vi "CmsInitializeQbus.vi"(8 "error in (no error)":errorcluster) -> (0 "error out":errorcluster, 3 "Qbus out":refnum<class "Qbus.lvclass">)   [LabVIEW 2017]
uses:
  <vilib>/addons/Qbus/Qbus.lvclass
  <vilib>/addons/BlinkProcess/BlinkProcess.lvlib
  <vilib>/addons/TimerProcess/TimerProcess.lvlib
  <vilib>/addons/InsightCM/Devices/Shared/Common/ServerComm/ServerComm.lvlib
  <vilib>/addons/InsightCM/Devices/Shared/Common/Trigger/Trigger.lvlib
  <vilib>/addons/InsightCM/Devices/Shared/Cms/CmsAnalysis/CmsAnalysis.lvlib
  <vilib>/addons/TraceLogger/TraceLogger.lvlib
  <vilib>/addons/InsightCM/Devices/Shared/Common/FileManager/FileManager.lvlib
  <vilib>/addons/InsightCM/Devices/Shared/Cms/CmsFpgaBitfileManager/CmsFpgaBitfileManager.lvlib
  <vilib>/addons/InsightCM/Devices/Shared/Common/Controller/Controller.lvlib
  <vilib>/addons/InsightCM/Devices/Shared/Common/DataAccumulator/DataAccumulator.lvlib
  <vilib>/addons/InsightCM/Devices/Shared/Common/DeviceHealth/DeviceHealth.lvlib
  <vilib>/addons/InsightCM/Devices/Shared/Common/SinglePointClock/SinglePointClock.lvlib
  <vilib>/addons/InsightCM/Devices/Shared/Cms/CmsVirtualChannel/CmsVirtualChannel.lvlib
  <vilib>/addons/InsightCM/Devices/Shared/Cms/CmsTestPanel/CmsTestPanel.lvlib
  <vilib>/addons/InsightCM/Devices/Shared/Common/ModbusMaster/ModbusMaster.lvlib
  <vilib>/addons/InsightCM/Devices/Shared/Cms/CmsDataEventCreator/CmsDataEventCreator.lvlib
  <vilib>/addons/InsightCM/Devices/Shared/Common/OpState/OpState.lvlib
  <vilib>/addons/InsightCM/Devices/Shared/Common/TrendAlarm/TrendAlarm.lvlib
  <vilib>/addons/InsightCM/Devices/Shared/Cms/CmsAnalysisHighRate/CmsAnalysisHighRate.lvlib
  <vilib>/addons/InsightCM/Devices/Shared/Cms/CmsAcquisition/CmsAcquisition.lvlib
  <vilib>/addons/InsightCM/Devices/Shared/Common/ScanEngine/ScanEngine.lvlib
  <vilib>/addons/InsightCM/Devices/Shared/Cms/CmsBurstMode/BurstMode.lvlib
  <vilib>/addons/InsightCM/Devices/Shared/Common/OPCUAClient/OPCUAClient.lvlib
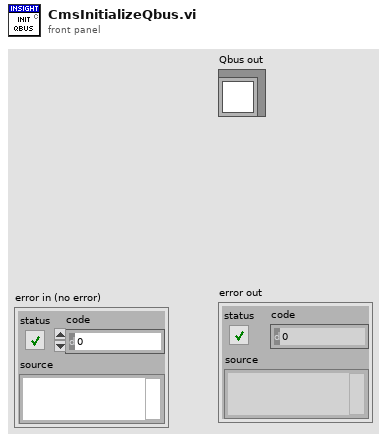
[diagram p1: front panel]
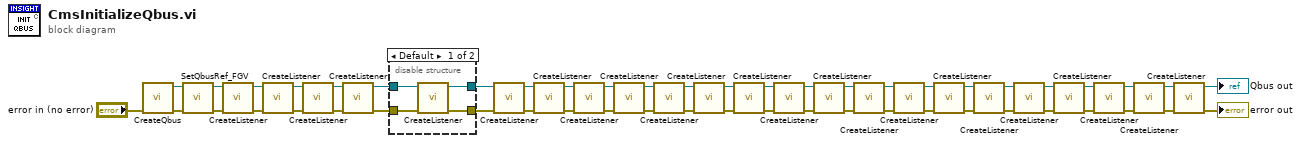
[diagram p0: block diagram]
diagram:
  n1 = call <vilib>:"CreateQbus.vi"("error in (no error)"="error in (no error)") -> ("error out"=w44:errorcluster, "Qbus"=w43:refnum<class "Qbus.lvclass">)  [unwired: 9 in]
  n2 = call <vilib>:"SetQbusRef_FGV.vi"("error in (no error)"=w44, "Qbus in"=w43) -> ("error out"=w42:errorcluster, "Qbus out"=w41:refnum<class "Qbus.lvclass">)  [unwired: 8 in]
  n3 = call <vilib>:"CreateListener.vi"("error in (no error)"=w42, "Qbus in"=w41) -> ("error out"=w46:errorcluster, "Qbus out"=w45:refnum<class "Qbus.lvclass">)  [unwired: 8 in]
  n4 = call <vilib>:"CreateListener.vi"("error in (no error)"=w46, "Qbus in"=w45) -> ("error out"=w33:errorcluster, "Qbus out"=w34:refnum<class "Qbus.lvclass">)  [unwired: 8 in]
  n5 = call <vilib>:"CreateListener.vi"("error in (no error)"=w33, "Qbus in"=w34) -> ("error out"=w32:errorcluster, "Qbus out"=w31:refnum<class "Qbus.lvclass">)  [unwired: 8 in]
  n6 = call <vilib>:"CreateListener.vi"("error in (no error)"=w32, "Qbus in"=w31) -> ("error out"=w2:errorcluster, "Qbus out"=w4:refnum<class "Qbus.lvclass">)  [unwired: 8 in]
  n7 = disable-structure shown="Default" {
    disable-tunnel: w4 -> [w55 w57]
    disable-tunnel: [w54 w57] -> w3
    disable-tunnel: w2 -> [w53 w56]
    disable-tunnel: [w52 w56] -> w1
    frame condition #0 (active) {
      n8 = call <vilib>:"CreateListener.vi"("error in (no error)"=w53, "Qbus in"=w55) -> ("error out"=w52:errorcluster, "Qbus out"=w54:refnum<class "Qbus.lvclass">)  [unwired: 8 in]
    }
    frame condition #1 {
    }
  }
  n9 = call <vilib>:"CreateListener.vi"("error in (no error)"=w1, "qbus in"=w3) -> ("error out"=w39:errorcluster, "qbus out"=w40:refnum<class "Qbus.lvclass">)  [unwired: 8 in]
  n10 = call <vilib>:"CreateListener.vi"("error in (no error)"=w39, "Qbus in"=w40) -> ("error out"=w29:errorcluster, "Qbus out"=w30:refnum<class "Qbus.lvclass">)  [unwired: 8 in]
  n11 = call <vilib>:"CreateListener.vi"("error in (no error)"=w29, "Qbus in"=w30) -> ("error out"=w28:errorcluster, "Qbus out"=w27:refnum<class "Qbus.lvclass">)  [unwired: 8 in]
  n12 = call <vilib>:"CreateListener.vi"("error in (no error)"=w28, "qbus in"=w27) -> ("error out"=w11:errorcluster, "qbus out"=w12:refnum<class "Qbus.lvclass">)  [unwired: 8 in]
  n13 = call <vilib>:"CreateListener.vi"("error in (no error)"=w11, "Qbus"=w12) -> ("error out"=w10:errorcluster, "Qbus out"=w13:refnum<class "Qbus.lvclass">)  [unwired: 8 in]
  n14 = call <vilib>:"CreateListener.vi"("error in (no error)"=w10, "qbus"=w13) -> ("error out"=w9:errorcluster, "qbus out"=w14:refnum<class "Qbus.lvclass">)  [unwired: 8 in]
  n15 = call <vilib>:"CreateListener.vi"("error in (no error)"=w9, "Qbus"=w14) -> ("error out"=w21:errorcluster, "Qbus out"=w22:refnum<class "Qbus.lvclass">)  [unwired: 8 in]
  n16 = call <vilib>:"CreateListener.vi"("error in (no error)"=w21, "Qbus"=w22) -> ("error out"=w20:errorcluster, "Qbus out"=w19:refnum<class "Qbus.lvclass">)  [unwired: 8 in]
  n17 = call <vilib>:"CreateListener.vi"("error in (no error)"=w20, "Qbus in"=w19) -> ("error out"=w24:errorcluster, "Qbus out"=w23:refnum<class "Qbus.lvclass">)  [unwired: 8 in]
  n18 = call <vilib>:"CreateListener.vi"("error in (no error)"=w24, "Qbus in"=w23) -> ("error out"=w7:errorcluster, "Qbus out"=w8:refnum<class "Qbus.lvclass">)  [unwired: 8 in]
  n19 = call <vilib>:"CreateListener.vi"("error in (no error)"=w7, "Qbus in"=w8) -> ("error out"=w6:errorcluster, "Qbus out"=w5:refnum<class "Qbus.lvclass">)  [unwired: 8 in]
  n20 = call <vilib>:"CreateListener.vi"("error in (no error)"=w6, "Qbus in"=w5) -> ("error out"=w26:errorcluster, "Qbus out"=w25:refnum<class "Qbus.lvclass">)  [unwired: 8 in]
  n21 = call <vilib>:"CreateListener.vi"("error in (no error)"=w26, "Qbus in"=w25) -> ("error out"=w38:errorcluster, "Qbus out"=w37:refnum<class "Qbus.lvclass">)  [unwired: 8 in]
  n22 = call <vilib>:"CreateListener.vi"("error in (no error)"=w38, "Qbus"=w37) -> ("error out"=w16:errorcluster, "Qbus out"=w15:refnum<class "Qbus.lvclass">)  [unwired: 8 in]
  n23 = call <vilib>:"CreateListener.vi"("error in (no error)"=w16, "Qbus in"=w15) -> ("error out"=w17:errorcluster, "Qbus out"=w18:refnum<class "Qbus.lvclass">)  [unwired: 8 in]
  n24 = call <vilib>:"CreateListener.vi"("error in (no error)"=w17, "Qbus in"=w18) -> ("error out"=w35:errorcluster, "Qbus out"=w36:refnum<class "Qbus.lvclass">)  [unwired: 8 in]
  n25 = call <vilib>:"CreateListener.vi"("error in (no error)"=w35, "Qbus in"=w36) -> ("error out"=w50:errorcluster, "Qbus out"=w51:refnum<class "Qbus.lvclass">)  [unwired: 8 in]
  n26 = call <vilib>:"CreateListener.vi"("error in (no error)"=w50, "qbus in"=w51) -> ("error out"=→"error out":errorcluster, "qbus out"=→"Qbus out":refnum<class "Qbus.lvclass">)  [unwired: 8 in]
